vi "OpenImageFile.vi"() -> ()   [LabVIEW 2017]
uses:
  <vilib>/vision/NI_Vision_Development_Module.lvlib
panel:
  out "Pixel Area":dbl
  in  "Blue or luminance":cluster{"Lower value":i32, "Upper value":i32}={"Lower value"=9, "Upper value"=93}
  in  "Green or saturation":cluster{"Lower value":i32, "Upper value":i32}={"Lower value"=148, "Upper value"=255}
  in  "Red or Hue":cluster{"Lower value":i32, "Upper value":i32}={"Lower value"=155, "Upper value"=245}
  out "Turn degrees":dbl
  out "Center of Mass X":dbl
  out "Original Image":T1(plugin-control)
  in  "File Path":path
  out "Apply Convex Hull":T1(plugin-control)
  # "This VI is for testing purposes"
  # "The Vision_Version_1 doesn't allow for opening a file anymore"
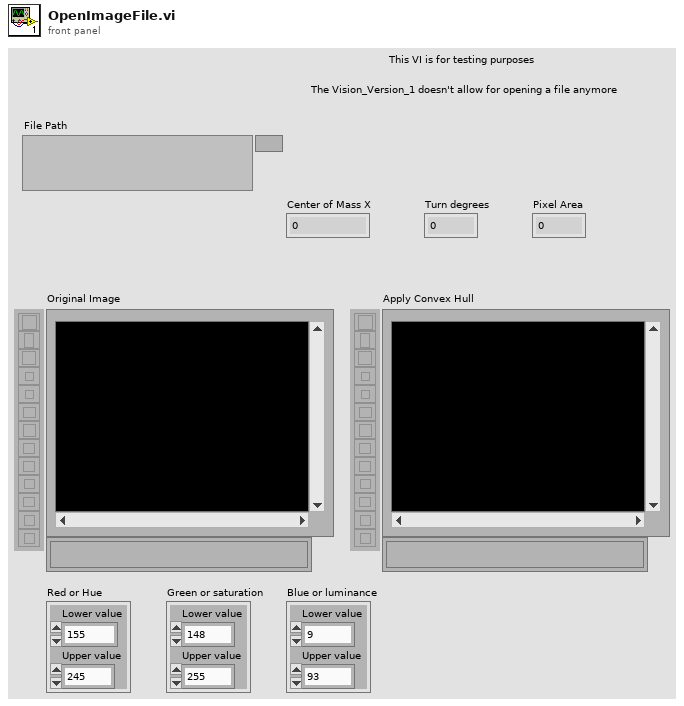
[diagram p1: front panel]
types:
  T1 = typedef "IMAQ Image.ctl" = refnum<image>
  T2 = typedef "Image Type" = u32
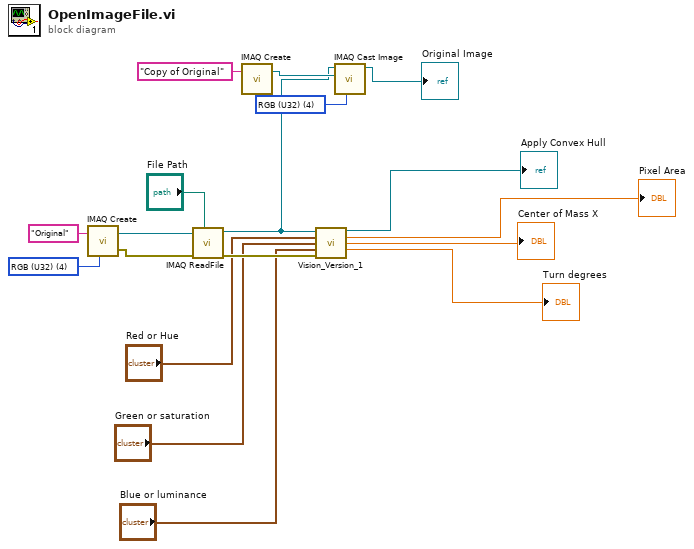
[diagram p0: block diagram]
diagram:
  w5 = T2 4 items=["Grayscale (U8)", "Grayscale (I16)", "Grayscale (SGL)", "Complex (CSG)", "RGB (U32)", "HSL (U32)", "RGB (U64)", "Grayscale (U16)"] ("Image Type")
  w10 = T2 4 items=["Grayscale (U8)", "Grayscale (I16)", "Grayscale (SGL)", "Complex (CSG)", "RGB (U32)", "HSL (U32)", "RGB (U64)", "Grayscale (U16)"] ("Image Type")
  n1 = call "IMAQ Create"("Image Name"="Original", "Image Type"=w10) -> ("New Image"=w17:T1, "error out"=w16:errorcluster)  [unwired: 3 in]
  n2 = call "IMAQ ReadFile"("File Path"="File Path", "error in (no error)"=w16, "Image"=w17) -> ("error out"=w15:errorcluster, "Image Out"=w7:T1)  [unwired: 4 in, 3 out]
  n3 = call "IMAQ Create"("Image Name"="Copy of Original") -> ("New Image"=w8:T1)  [unwired: 4 in, 1 out]
  n4 = call "Vision_Version_1.vi"("Source Image"=w7, "Red or Hue"="Red or Hue", "Green or saturation"="Green or saturation", "Blue or luminance"="Blue or luminance", "Error in"=w15) -> ("Apply Convex Hull"=→"Apply Convex Hull":T1, "Pixel Area"=→"Pixel Area":dbl, "Center of Mass X"=→"Center of Mass X":dbl, "Turn degrees"=→"Turn degrees":dbl)  [unwired: 5 in, 2 out]
  n5 = call "IMAQ Cast Image"("Image Type"=w5, "Image Dst"=w8, "Image Src"=w7) -> ("Image Dst Out"=→"Original Image":T1)  [unwired: 7 in, 1 out]
